vi "sub_main_speed-control.vi"(8 "error in":errorcluster) -> (0 "error out":errorcluster)   [LabVIEW 2019]
uses:
  Ctrl/obstacle_info.ctl
  Ctrl/cmd_common.ctl
  Ctrl/pid-in-params.ctl
  Ctrl/agv_cmd_v.ctl
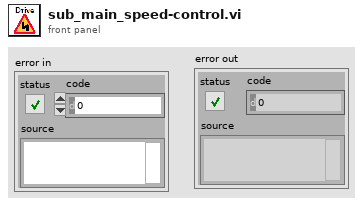
[diagram p1: front panel]
types:
  T1 = typedef "obstacle_info.ctl" = enum16{"init", "read", "obstacle status in", "write limit", "inrange pt-n"}
  T2 = typedef "agv_cmd_v.ctl" = enum16{"write limit", "init stop", "write", "read"}
  T3 = typedef "cmd_common.ctl" = enum16{"read", "write"}
  T4 = typedef "pid-in-params.ctl" = enum16{"read", "write"}
  T5 = typedef "state.ctl" = enum16{"init", "Test circular track", "start point", "start heading adjust", "wait before start", "stop point check", "stop point start", "end point", "entering ending point", "move", "move heading adjust"}
  T6 = cluster{" turn angular speed":dbl, "move linear speed":dbl, "decrease factor linear speed":dbl, "adjust angle margin":dbl}
  T7 = cluster{"v_linear":dbl, " turn angular speed":dbl}
  T8 = cluster{"deg_agv-lookahead":dbl, "deg_waypoint":dbl, "deg_gap":dbl, "deg_target":dbl, "pid output":dbl, "dis-gap":dbl, "deg_agv-center":dbl}
  T9 = cluster{"Port":refnum<visa-resource-name>, "limits":cluster{"speed limits":cluster{"max":dbl, "min":dbl}, "steer limits":cluster{"max":dbl, "min":dbl}}}
  T10 = typedef "system_hw.ctl" = cluster{"AGV":enum16{"none", "ERP42", "ERP42mini", "Scout", "Ycar"}, "Lidar 1":enum16{"none", "VLP16", "TIM571", "RPLidar A2", "RPLidar A3"}, "Lidar 2":enum16{"none", "VLP16", "TIM571", "RPLidar A2", "RPLidar A3"}, "GPS":enum16{"none", "F9P", "M8P", "PwrPak7", "19X HVS"}, "Camera":enum16{"none", "C920", "C922", "GT1290C", "MS LifeCam"}, "Joystick":enum16{"none", "joystick"}, "sound":enum16{"none", "speaker"}, "IMU":enum16{"none", "MW-AHRSv1"}}
  T11 = enum16{"none", "ERP42", "ERP42mini", "Scout", "Ycar"}
  T12 = typedef "data.ctl" = cluster{"Drive_value":cluster{"F/B":enum16{"Go", "N", "Back"}, "Speed":u16, "Steer":i16, "A/M":enum16{"Brake", "Auto", "Manual"}, "Brake":u8}}
  T13 = typedef "joystick cfg.ctl" = cluster{"Type":enum16{"Logitech F710", "Xbox"}, "steer limit":cluster{"min":dbl, "max":dbl, "scale":dbl, "offset":dbl}, "speed limit":cluster{"min":dbl, "max":dbl, "pwm max":dbl}, "ID":i32, "joystick max":dbl}
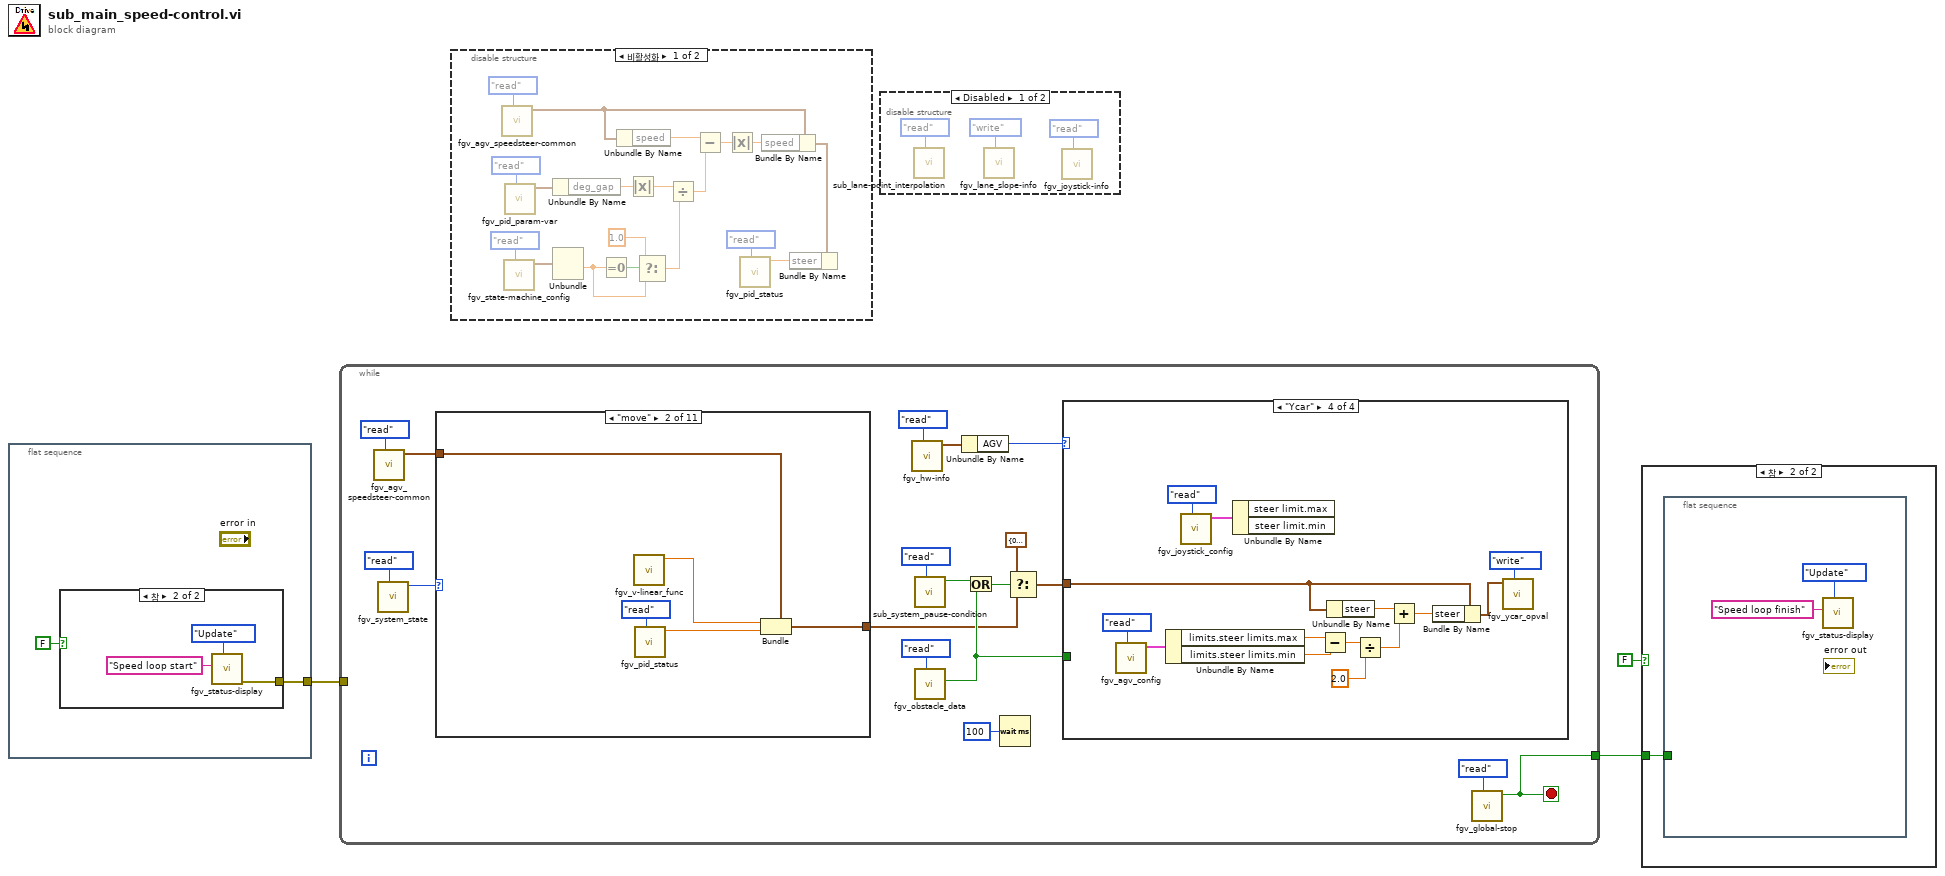
[diagram p0: block diagram]
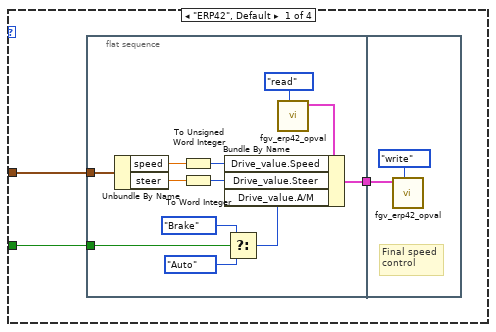
[diagram p6: hidden frame]
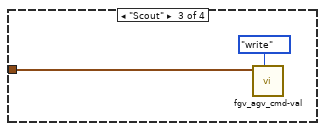
[diagram p8: hidden frame]
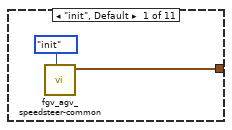
[diagram p9: hidden frame]
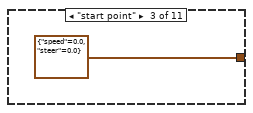
[diagram p10: hidden frame]
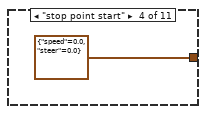
[diagram p11: hidden frame]
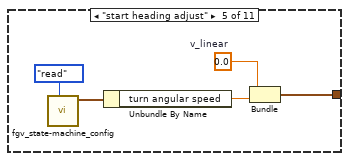
[diagram p12: hidden frame]
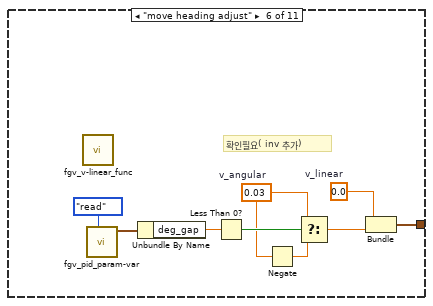
[diagram p13: hidden frame]
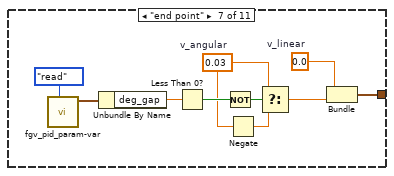
[diagram p14: hidden frame]
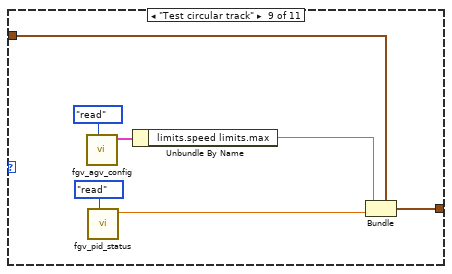
[diagram p16: hidden frame]
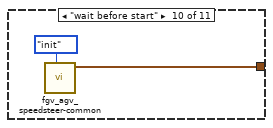
[diagram p17: hidden frame]
diagram:
  n1 = flat-sequence {
    tunnel: [w5] -> w3
    frame #0 {
      n2 = case shown="참" FALSE {
        tunnel: [_ w6] -> w5
        frame False {
        }
        frame True {
          n3 = call "fgv_status-display.vi"("Mode"=enum16{"Initial", "Update", "Clear"}."Update", "title"="Speed loop start" ("String in 1")) -> ("error out"=w6:errorcluster)  [unwired: 9 in]
        }
      }
    }
  }
  n4 = while {
    tunnel: w3 -> [_]
    tunnel: [w15] -> w2
    stop <- w15 stop-if-true
    n5 = call "fgv_agv_speedsteer-common.vi"("cmd"=enum16{"init", "read", "write"}."read") -> ("speed-steer out"=w12:cluster{"speed":dbl, "steer":dbl})  [unwired: 9 in, 1 out]
    n6 = call "fgv_system_state.vi"("cmd"=enum16{"init", "read", "write"}."read") -> ("State out"=w18:T5)  [unwired: 9 in, 1 out]
    n7 = case shown="\"move\"" w18 {
      tunnel: [w60 w62 cluster{"speed":dbl, "steer":dbl} {"speed"=0.0, "steer"=0.0} ("t") cluster{"speed":dbl, "steer":dbl} {"speed"=0.0, "steer"=0.0} ("t") w72 w74 w83 _ w98 w100 w102] -> w9
      tunnel: w12 -> [_ w63 _ _ _ _ _ _ w94 _ w102]
      frame "init", Default {
        n8 = call "fgv_agv_speedsteer-common.vi"("cmd"=enum16{"init", "read", "write"}."init") -> ("speed-steer out"=w60:cluster{"speed":dbl, "steer":dbl})  [unwired: 9 in, 1 out]
      }
      frame "move" {
        n9 = call "fgv_v-linear_func.vi"() -> ("velocity_out"=w65:dbl)  [unwired: 11 in]
        n10 = call "fgv_pid_status.vi"("cmd"=cmd_common."read") -> ("pid output"=w64:dbl)  [unwired: 8 in, 2 out]
        n11 = Bundle(cluster=w63, "speed"=w65, "steer"=w64) -> (w62:cluster{"speed":dbl, "steer":dbl})
      }
      frame "start point" {
      }
      frame "stop point start" {
      }
      frame "start heading adjust" {
        w73 = 0.0  # v_linear
        n12 = call "fgv_state-machine_config.vi"("cmd"=enum16{"write", "read"}."read") -> ("Angle cfg out"=w70:T6)  [unwired: 10 in]
        n13 = Unbundle By Name(w70) -> ("turn angular speed"=w69:dbl)
        n14 = Bundle("v_linear"=w73, "turn angular speed"=w69) -> (w72:T7)  [unwired: 1 in]
      }
      frame "move heading adjust" {
        w77 = 0.0  # v_linear
        w76 = 0.03  # v_angular
        # "확인필요( inv 추가)"
        n15 = call "fgv_v-linear_func.vi"() -> ()  [unwired: 11 in, 1 out]
        n16 = call "fgv_pid_param-var.vi"("cmd"=pid-in-params."read") -> ("pid-var_output"=w78:T8)  [unwired: 10 in]
        n17 = Unbundle By Name(w78) -> ("deg_gap"=w80:dbl)
        n18 = Less Than 0?(x=w80) -> (x < 0?=w81:bool)
        n19 = Negate(x=w76) -> (-x=w79:dbl)
        n20 = Select(t=w76, s=w81, f=w79) -> (s? t:f=w82:dbl)
        n21 = Bundle("v_linear"=w77, "v_angular"=w82) -> (w74:cluster{"v_linear":dbl, "v_angular":dbl})  [unwired: 1 in]
      }
      frame "end point" {
        w86 = 0.0  # v_linear
        w85 = 0.03  # v_angular
        n22 = call "fgv_pid_param-var.vi"("cmd"=pid-in-params."read") -> ("pid-var_output"=w87:T8)  [unwired: 10 in]
        n23 = Unbundle By Name(w87) -> ("deg_gap"=w89:dbl)
        n24 = Less Than 0?(x=w89) -> (x < 0?=w90:bool)
        n25 = Not(x=w90) -> (.not. x?=w91:bool)
        n26 = Negate(x=w85) -> (-x=w88:dbl)
        n27 = Select(t=w85, s=w91, f=w88) -> (s? t:f=w92:dbl)
        n28 = Bundle("v_linear"=w86, "v_angular"=w92) -> (w83:cluster{"v_linear":dbl, "v_angular":dbl})  [unwired: 1 in]
      }
      frame "entering ending point" {
      }
      frame "Test circular track" {
        n29 = call "fgv_agv_config.vi"("cmd"=enum16{"read", "write"}."read") -> ("AGV cfg out"=w96:T9)  [unwired: 9 in, 1 out]
        n30 = call "fgv_pid_status.vi"("cmd"=cmd_common."read") -> ("pid output"=w99:dbl)  [unwired: 8 in, 2 out]
        n31 = Unbundle By Name(w96) -> ("limits.speed limits.max"=w95:dbl)
        n32 = Bundle(cluster=w94, "speed"=w95, "steer"=w99) -> (w98:cluster{"speed":dbl, "steer":dbl})
      }
      frame "wait before start" {
        n33 = call "fgv_agv_speedsteer-common.vi"("cmd"=enum16{"init", "read", "write"}."init") -> ("speed-steer out"=w100:cluster{"speed":dbl, "steer":dbl})  [unwired: 9 in, 1 out]
      }
      frame "stop point check" {
      }
    }
    n34 = call "fgv_hw-info.vi"("cmd"=enum16{"write", "read"}."read") -> ("HW info out"=w11:T10)  [unwired: 10 in]
    n35 = call "sub_system_pause-condition.vi"("cmd"=enum16{"pause", "go", "read"}."read") -> ("pause"=w17:bool)  [unwired: 10 in]
    n36 = call "fgv_obstacle_data.vi"("cmd"=obstacle_info."read") -> ("obstacle out"=w16:bool)  [unwired: 7 in, 3 out]
    n37 = Unbundle By Name(w11) -> ("AGV"=w10:T11)
    n38 = Or(x=w17, y=w16) -> (x .or. y?=w19:bool)
    n39 = Wait (ms)(milliseconds to wait=u32 100) -> ()  [unwired: 1 out]
    n40 = Select(t=cluster{"speed":dbl, "steer":dbl} {"speed"=0.0, "steer"=0.0}, s=w19, f=w9) -> (s? t:f=w21:cluster{"speed":dbl, "steer":dbl})
    n41 = case shown="\"Ycar\"" w10 {
      tunnel: w21 -> [w28 _ w44 w49]
      tunnel: w16 -> [w27 _ _ _]
      frame "ERP42", Default {
        n42 = flat-sequence {
          tunnel: w28 -> [w39]
          tunnel: w27 -> [w32]
          tunnel: [w31] -> w29
          tunnel: w29 -> [w42]
          frame #0 {
            n43 = Unbundle By Name(w39) -> ("speed"=w37:dbl, "steer"=w38:dbl)
            n44 = To Unsigned Word Integer(number=w37) -> (unsigned 16bit integer=w36:u16)
            n45 = To Word Integer(number=w38) -> (16bit integer=w35:i16)
            n46 = Select(t=enum16{"Brake", "Auto", "Manual"}."Brake" ("Drive_value.A/M"), s=w32, f=enum16{"Brake", "Auto", "Manual"}."Auto" ("Drive_value.A/M")) -> (s? t:f=w30:enum16{"Brake", "Auto", "Manual"})
            n47 = call "fgv_erp42_opval.vi"("cmd"=enum16{"read", "write", "ini"}."read") -> ("data_out"=w40:T12)  [unwired: 10 in]
            n48 = Bundle By Name(cluster=w40, "Drive_value.Speed"=w36, "Drive_value.Steer"=w35, "Drive_value.A/M"=w30) -> (w31:T12)
          }
          frame #1 {
            # "Final speed\ncontrol"
            n49 = call "fgv_erp42_opval.vi"("cmd"=enum16{"read", "write", "ini"}."write", "data_in"=w42) -> ()  [unwired: 9 in, 1 out]
          }
        }
      }
      frame "ERP42mini" {
      }
      frame "Scout" {
        n50 = call "fgv_agv_cmd-val.vi"("cmd"=agv_cmd_v."write", "agv_speed_in"=w44) -> ()  [unwired: 8 in, 2 out]
      }
      frame "Ycar" {
        n51 = call "fgv_agv_config.vi"("cmd"=enum16{"read", "write"}."read") -> ("AGV cfg out"=w58:T9)  [unwired: 9 in, 1 out]
        n52 = Unbundle By Name(w58) -> ("limits.steer limits.max"=w47:dbl, "limits.steer limits.min"=w46:dbl)
        n53 = call "fgv_joystick_config.vi"("cmd"=cmd_common."read") -> ("Joystick cfg out"=w55:T13)  [unwired: 9 in, 1 out]
        n54 = Unbundle By Name(w55) -> ()  [unwired: 2 out]
        n55 = Subtract(x=w47, y=w46) -> (x-y=w56:dbl)
        n56 = Unbundle By Name(w49) -> ("steer"=w51:dbl)
        n57 = Divide(x=w56, y=2.0) -> (x/y=w52:dbl)
        n58 = Add(x=w51, y=w52) -> (x+y=w50:dbl)
        n59 = Bundle By Name(cluster=w49, "steer"=w50) -> (w48:cluster{"speed":dbl, "steer":dbl})
        n60 = call "fgv_ycar_opval.vi"("cmd"=enum16{"read", "write", "ini"}."write", "opval"=w48) -> ()  [unwired: 9 in, 1 out]
      }
    }
    n61 = call "fgv_global-stop.vi"("cmd"=enum16{"init", "stop", "read"}."read") -> ("val_out"=w15:bool)  [unwired: 10 in]
  }
  n62 = disable-structure shown="비활성화" {
    frame Disabled {
      n63 = call "fgv_agv_speedsteer-common.vi"("cmd"=enum16{"init", "read", "write"}."read") -> ("speed-steer out"=w103:cluster{"speed":dbl, "steer":dbl})  [unwired: 9 in, 1 out]
      n64 = call "fgv_state-machine_config.vi"("cmd"=enum16{"write", "read"}."read") -> ("Angle cfg out"=w108:T6)  [unwired: 10 in]
      n65 = call "fgv_pid_param-var.vi"("cmd"=pid-in-params."read") -> ("pid-var_output"=w107:T8)  [unwired: 10 in]
      n66 = Unbundle By Name(w107) -> ("deg_gap"=w109:dbl)
      n67 = Unbundle(w108) -> ("decrease factor linear speed"=w117:dbl)  [unwired: 3 out]
      n68 = Equal To 0?(x=w117) -> (x = 0?=w116:bool)
      n69 = Unbundle By Name(w103) -> ("speed"=w113:dbl)
      n70 = Absolute Value(x=w109) -> (abs(x)=w121:dbl)
      n71 = Select(t=1.0, s=w116, f=w117) -> (s? t:f=w119:dbl)
      n72 = Divide(x=w121, y=w119) -> (x/y=w112:dbl)
      n73 = Subtract(x=w113, y=w112) -> (x-y=w114:dbl)
      n74 = Absolute Value(x=w114) -> (abs(x)=w120:dbl)
      n75 = call "fgv_pid_status.vi"("cmd"=cmd_common."read") -> ("pid output"=w106:dbl)  [unwired: 8 in, 2 out]
      n76 = Bundle By Name(cluster=w103, "speed"=w120) -> (w115:cluster{"speed":dbl, "steer":dbl})
      n77 = Bundle By Name(cluster=w115, "steer"=w106) -> ()  [unwired: 1 out]
    }
    frame Enabled {
    }
  }
  n78 = disable-structure shown="Disabled" {
    frame Disabled {
      n79 = call "sub_lane-point_interpolation.vi"("cmd"=enum16{"init", "read", "write"}."read") -> ()  [unwired: 7 in, 4 out]
      n80 = call "fgv_lane_slope-info.vi"("cmd"=enum16{"ini", "read", "write"}."write") -> ()  [unwired: 8 in, 3 out]
      n81 = call "fgv_joystick-info.vi"("init"=enum16{"enable", "init", "read", "write"}."read") -> ()  [unwired: 7 in, 4 out]
    }
    frame Enabled {
    }
  }
  n82 = case shown="참" FALSE {
    tunnel: w2 -> [_ w125]
    frame False {
    }
    frame True {
      n83 = flat-sequence {
        tunnel: w125 -> [_]
        frame #0 {
          n84 = call "fgv_status-display.vi"("Mode"=enum16{"Initial", "Update", "Clear"}."Update", "title"="Speed loop finish" ("String in 1")) -> ()  [unwired: 9 in, 1 out]
        }
      }
    }
  }
